vi "process.vi"(8 "error in":errorcluster, 10 "state":string, 11 "process in":string) -> (0 "error out":errorcluster, 2 "process out":string)   [LabVIEW 2016]
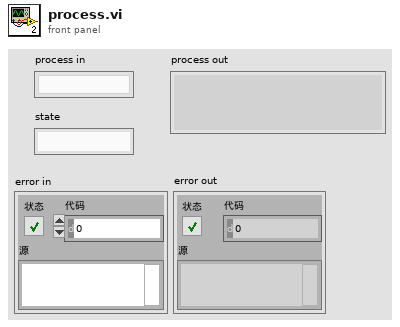
[diagram p1: front panel]
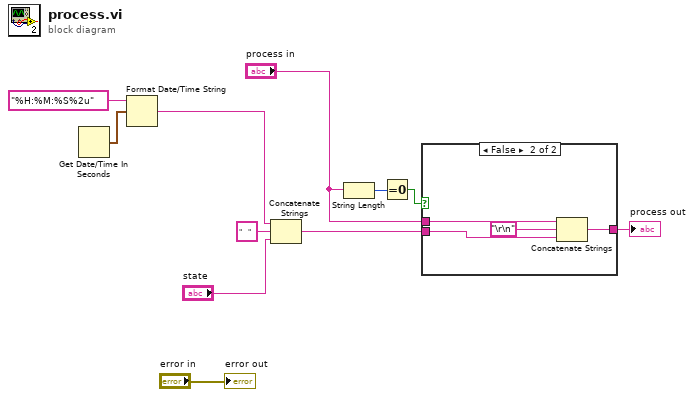
[diagram p0: block diagram]
diagram:
  n1 = Get Date/Time In Seconds() -> (seconds since 1Jan1904=w4:timestamp)
  n2 = Format Date/Time String(time format string (%c)="%H:%M:%S%2u", seconds (now)=w4) -> (date/time string=w2:string)  [unwired: 1 in]
  n3 = Concatenate Strings(w2, "   " ("字符串"), "state") -> (w9:string)
  n4 = String Length(string="process in") -> (length=w6:i32)
  n5 = Equal To 0?(x=w6) -> (x = 0?=w5:bool)
  n6 = case shown="False" w5 {
    tunnel: w9 -> [w12 w16]
    tunnel: [w12 w15] -> w8
    tunnel: "process in" -> [_ w13]
    frame True {
    }
    frame False {
      n7 = Concatenate Strings(w13, "\r\n", w16) -> (w15:string)
    }
  }
  "process out" <- w8
  "error out" <- "error in"
